vi "SwissSPAD Live_Get-Set Histogram Cursor Locations.vi"(6 "Get (F)/Set":bool, 8 "Error In":errorcluster, 10 "X":dbl, 11 "CursIdx":i32) -> (0 "Error Out":errorcluster, 1 "Histogram Cursor Locations":cluster{"Min Cursor":dbl, "Max Cursor":dbl}, 2 "X":dbl)   [LabVIEW 2021]
uses:
  SwissSPAD Live_Internal Data List.ctl
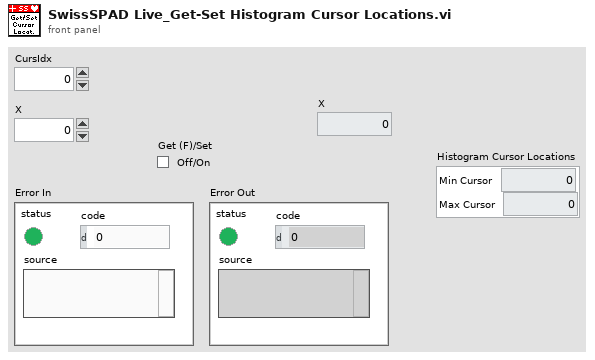
[diagram p1: front panel]
types:
  T1 = typedef "SwissSPAD Live_Internal Data List.ctl" = enum16{"Number of pending file saving tasks", "File Saving Tasks Information", "Current Image ROI Information", "# FPGA Reset Attempts", "Histogram Cursor Locations", "Histogram Window is Open"}
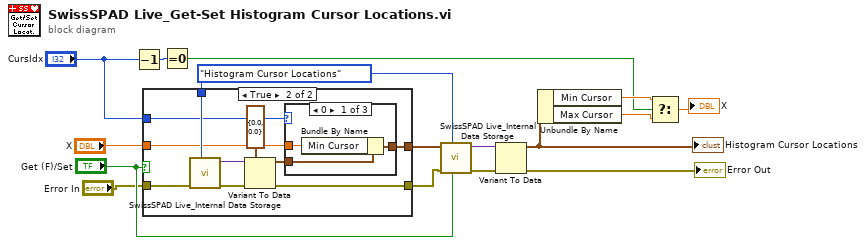
[diagram p0: block diagram]
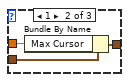
[diagram p3: hidden frame]
diagram:
  w7 = SwissSPAD_Live_Internal_Data_List."Histogram Cursor Locations" ("SS2 Live Data")
  n1 = Decrement(x="CursIdx") -> (x-1=w6:i32)
  n2 = case shown="True" "Get (F)/Set" {
    tunnel: w7 -> [_ w27]
    tunnel: "CursIdx" -> [_ w23]
    tunnel: "X" -> [_ w21]
    tunnel: [_ w20] -> w4
    tunnel: "Error In" -> [w17 w19]
    tunnel: [w17 w18] -> w2
    frame False {
    }
    frame True {
      n3 = call "SwissSPAD Live_Internal Data Storage.vi"("SS2 Live Data"=w27, "Error In"=w19) -> ("Error Out"=w25:errorcluster, "Variant"=w26:variant)  [unwired: 7 in, 1 out]
      n4 = Variant To Data(error in=w25, type=cluster{"Min Cursor":dbl, "Max Cursor":dbl} {"Min Cursor"=0.0, "Max Cursor"=0.0} ("Histogram Cursor Locations"), Variant=w26) -> (data=w22:cluster{"Min Cursor":dbl, "Max Cursor":dbl}, error out=w18:errorcluster)
      n5 = case shown="0" w23 {
        tunnel: w22 -> [w30 w33 w34]
        tunnel: w21 -> [w29 w32 _]
        tunnel: [w28 w31 w34] -> w20
        frame 0 {
          n6 = Bundle By Name(cluster=w30, "Min Cursor"=w29) -> (w28:cluster{"Min Cursor":dbl, "Max Cursor":dbl})
        }
        frame 1 {
          n7 = Bundle By Name(cluster=w33, "Max Cursor"=w32) -> (w31:cluster{"Min Cursor":dbl, "Max Cursor":dbl})
        }
        frame 2, Default {
        }
      }
    }
  }
  n8 = Equal To 0?(x=w6) -> (x = 0?=w10:bool)
  n9 = call "SwissSPAD Live_Internal Data Storage.vi"("Get(F)/Set"="Get (F)/Set", "SS2 Live Data"=w7, "Error In"=w2, "Variant"=w4) -> ("Error Out"=w15:errorcluster, "Variant"=w16:variant)  [unwired: 5 in, 1 out]
  n10 = Variant To Data(error in=w15, Variant=w16) -> (data=w13:cluster{"Min Cursor":dbl, "Max Cursor":dbl}, error out=→"Error Out":errorcluster)  [unwired: 1 in]
  "Histogram Cursor Locations" <- w13
  n11 = Unbundle By Name(w13) -> ("Min Cursor"=w12:dbl, "Max Cursor"=w11:dbl)
  n12 = Select(t=w12, s=w10, f=w11) -> (s? t:f=→"X":dbl)
